vi "Demo.vi"(8 "error in":errorcluster) -> (0 "error out":errorcluster)   [LabVIEW 2024, in "Application.lvlib"]
uses:
  Application.lvlib
  Modules/User Interface/User Interface.lvlib
  Modules/Session Scanner/Session Scanner.lvlib
  Modules/Data Base/Data Base.lvlib
  Modules/Error Handler/Error Handler.lvlib
panel:
  # "Hardware Seeker Tool"
  # "DEMO"
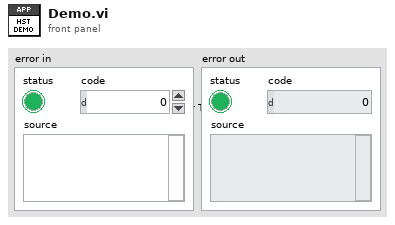
[diagram p1: front panel]
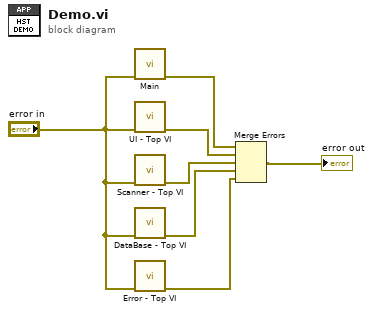
[diagram p0: block diagram]
diagram:
  n1 = call "Main.vi"("error in"="error in") -> ("error out"=w6:errorcluster)  [unwired: 10 in]
  n2 = call "UI - Top VI.vi"("error in"="error in") -> ("error out"=w5:errorcluster)  [unwired: 10 in]
  n3 = call "Scanner - Top VI.vi"("error in"="error in") -> ("error out"=w4:errorcluster)  [unwired: 10 in]
  n4 = call "DataBase - Top VI.vi"("error in"="error in") -> ("error out"=w3:errorcluster)  [unwired: 10 in]
  n5 = call "Error - Top VI.vi"("error in"="error in") -> ("error out"=w2:errorcluster)  [unwired: 10 in]
  n6 = Merge Errors(w6, w5, w4, w3, w2) -> (→"error out":errorcluster)
